vi "Fuzzy Controller.vi"(3 "Controller data":T1 {"Parameters"."defu"."defaultvalue" format="%.2f"; "Parameters"."degree-of-support" step=0.009999999776482582 format="%.2f"; "Parameters"."consequence"."x-min" step=0.009999999776482582 format="%.2f"; "Parameters"."consequence"."x-max" step=0.009999999776482582 format="%.2f"; "Parameters"."consequence"."setarray"."points" step=0.009999999776482582 format="%.2f"; "Parameters"."antecedance"."x-min" step=0.009999999776482582 format="%.2f"; "Parameters"."antecedance"."x-max" step=0.009999999776482582 format="%.2f"; "Parameters"."antecedance"."setarray"."points" step=0.009999999776482582 format="%.2f"}, 4 "in4":dbl format="%.2f", 5 "name 1":string, 6 "name 4":string, 7 "in1":dbl step=0.01 format="%.2f", 8 "in3":dbl format="%.2f", 9 "name 3":string, 10 "in2":dbl format="%.2f", 11 "name 2":string) -> (0 "error-array":errorcluster[](array[cluster]), 1 "output assessment":string="last result", 2 "analog output":dbl format="%.2f")   [LabVIEW 2020, in "NI_fuzzy logic.lvlib"]
doc: "LabVIEW no longer supports this VI.\nThis VI is implements a Fuzzy Logic Controller. A controller data file (the project file generated by the Fuzzy Logic Controller Design Project Manager) needs to be loaded by the Load Fuzzy Controller VI."
uses:
  <vilib>/addons/control/fuzzy/NI_fuzzy logic.lvlib
  <vilib>/addons/control/fuzzy/fuzzy logic.llb/Fuzzy Datatype.ctl
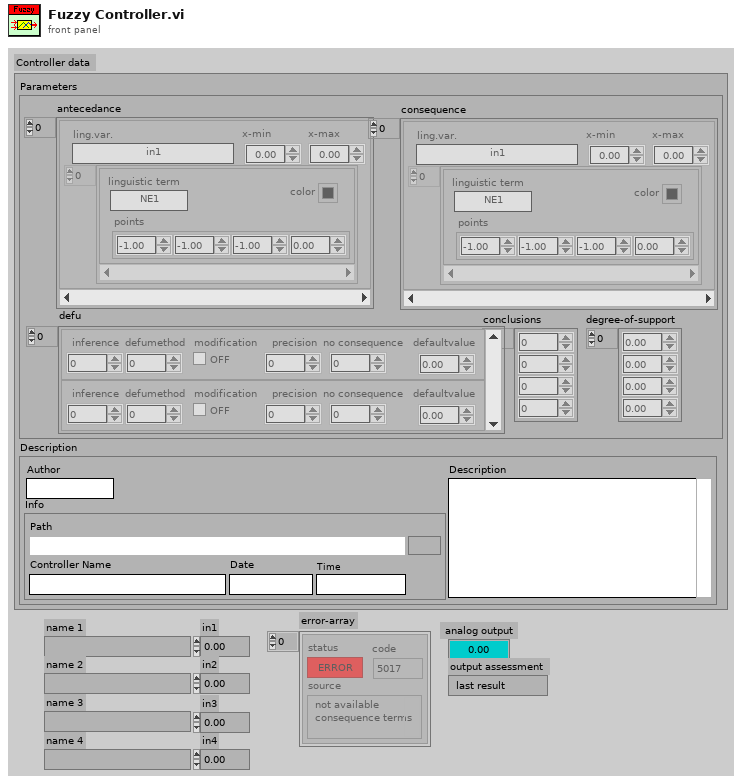
[diagram p1: front panel]
types:
  T1 = typedef "NI_fuzzy logic.lvlib/Fuzzy Datatype.ctl" = cluster{"Parameters":cluster{"antecedance":cluster{"ling.var.":string, "x-min":dbl, "x-max":dbl, "setarray":cluster{"linguistic term":string, "color":u32, "points":dbl[]}[]}[], "consequence":cluster{"ling.var.":string, "x-min":dbl, "x-max":dbl, "setarray":cluster{"linguistic term":string, "color":u32, "points":dbl[]}[]}[], "conclusions":u16[], "degree-of-support":dbl[], "defu":cluster{"inference":u16, "defumethod":u16, "modification":bool, "precision":u16, "no consequence":u16, "defaultvalue":dbl}[]}, "Description":cluster{"Info":cluster{"Path":path, "Controller Name":string, "Date":string, "Time":string}, "Author":string, "Description":string}}
  T2 = cluster{"index":i32, "fulfillment":dbl[], "active sets":i32[]}
  T3 = cluster{"fullfilment*DoS":dbl[], "active consequence":i32[]}
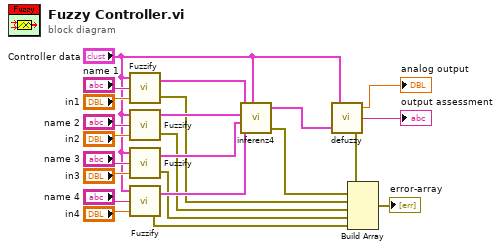
[diagram p0: block diagram]
diagram:
  n1 = call <vilib>:"Fuzzify.vi"("input-value"="in1", "input-name"="name 1", "Controller"="Controller data") -> ("error out"=w17:errorcluster, "fuzzified antecedance"=w18:T2)
  n2 = call <vilib>:"Fuzzify.vi"("input-value"="in2", "input-name"="name 2", "Controller"="Controller data") -> ("error out"=w16:errorcluster, "fuzzified antecedance"=w19:T2)
  n3 = call <vilib>:"Fuzzify.vi"("input-value"="in3", "input-name"="name 3", "Controller"="Controller data") -> ("error out"=w15:errorcluster, "fuzzified antecedance"=w21:T2)
  n4 = call <vilib>:"Fuzzify.vi"("input-value"="in4", "input-name"="name 4", "Controller"="Controller data") -> ("error out"=w14:errorcluster, "fuzzified antecedance"=w20:T2)
  n5 = call <vilib>:"inferenz4.vi"("fuzzified input 1"=w18, "fuzzified input 2"=w19, "fuzzified input 3"=w21, "fuzzified input 4"=w20, "Controller"="Controller data") -> ("fuzzified consequence"=w22:T3, "error out"=w23:errorcluster)  [unwired: 1 out]
  n6 = call <vilib>:"defuzzy.vi"("Controller"="Controller data", "inference results"=w22) -> ("analog output"=→"analog output":dbl, "output assessment"=→"output assessment":string, "error out"=w13:errorcluster)
  n7 = Build Array(w13, w23, w17, w16, w15, w14) -> (→"error-array":errorcluster[])
